vi "ConfMappIn.vi"(8 "error in (no error)":errorcluster, 11 "ConfMap In":string[](array[string])) -> (0 "error out":errorcluster, 1 "Discard?":bool, 3 "ConfMap Out":string[](array[string]))   [LabVIEW 2014, in "SeqLoop.lvlib"]
uses:
  SeqLoop.lvlib
panel:
  in  "Habilitada":bool
  in  "Bit":i32
  in  "Nro. Hardware":i32
  in  "Stop Med":bool
  in  "Add Med":bool
  in  "Descripción":string
  in  "Nro.":i32
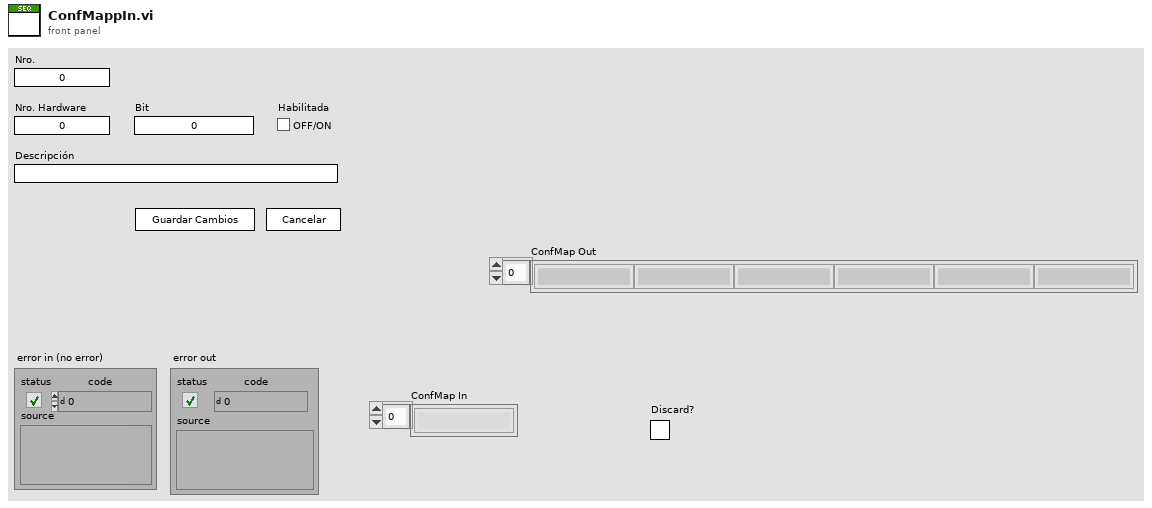
[diagram p1: front panel]
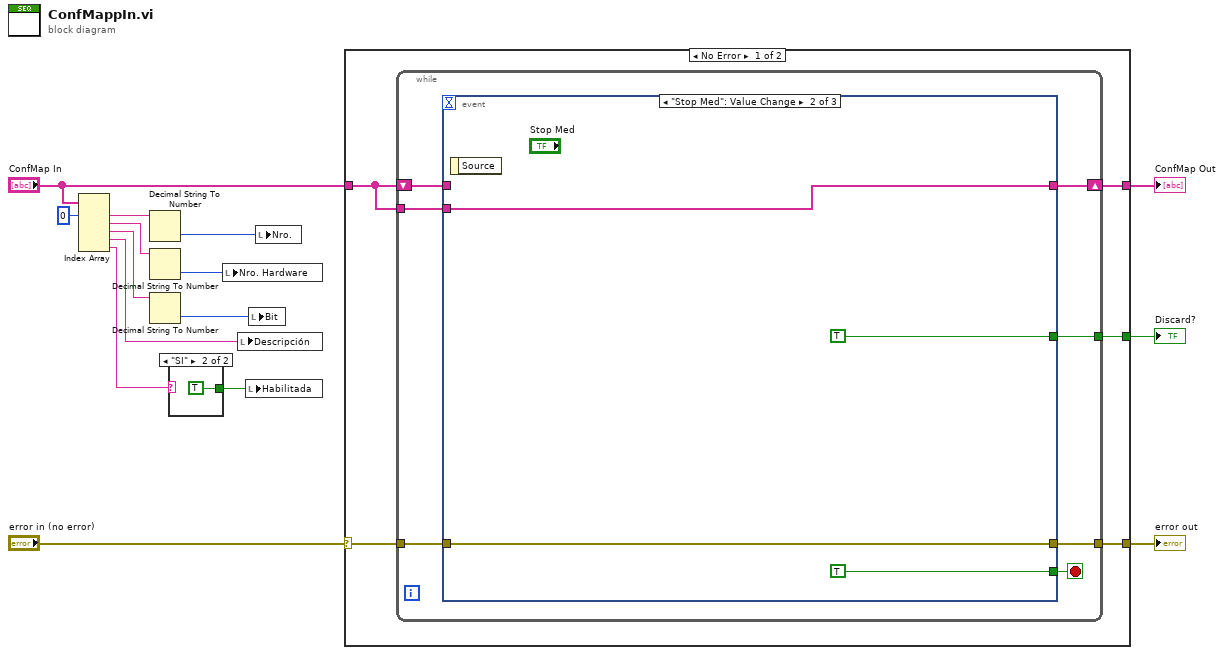
[diagram p0: block diagram]
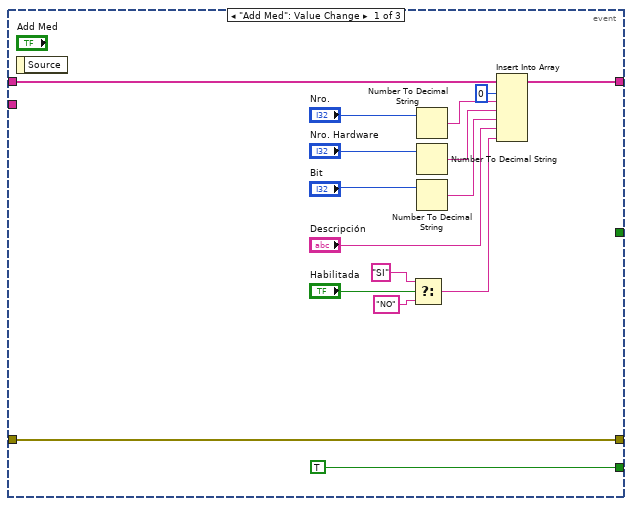
[diagram p3: hidden frame]
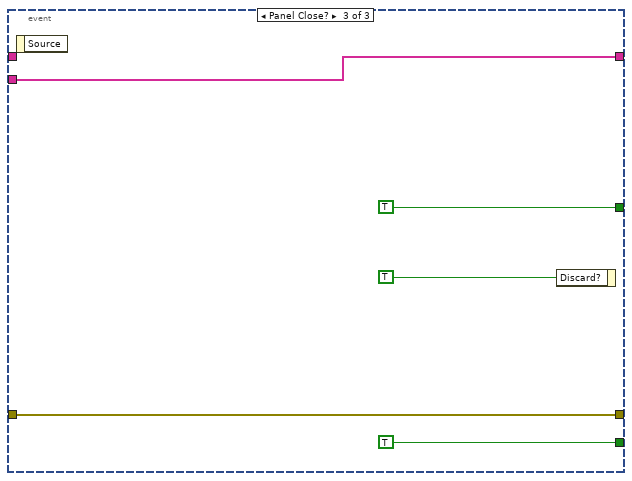
[diagram p4: hidden frame]
diagram:
  n1 = Index Array(array="ConfMap In", index #1=0 ("index")) -> (element #1=w10:string, element #2=w5:string, element #3=w4:string, element #4=w6:string, element #5=w3:string)  [unwired: 4 in]
  n2 = Decimal String To Number(string=w10) -> (number=w9:i32)  [unwired: 2 in, 1 out]
  n3 = Decimal String To Number(string=w5) -> (number=w8:i32)  [unwired: 2 in, 1 out]
  n4 = Decimal String To Number(string=w4) -> (number=w7:i32)  [unwired: 2 in, 1 out]
  n5 = case shown="\"SI\"" w3 {
    tunnel: [_ TRUE] -> w2
    frame "NO", Default {
    }
    frame "SI" {
    }
  }
  n6 = local write "Nro. Hardware"(w8) -> ()
  n7 = local write "Descripción"(w6) -> ()
  n8 = local write "Habilitada"(w2) -> ()
  n9 = local write "Bit"(w7) -> ()
  n10 = local write "Nro."(w9) -> ()
  n11 = case shown="No Error" "error in (no error)" {
    selector: "error in (no error)" -> [w19 w55]
    tunnel: [w21 w55] -> w14
    tunnel: "ConfMap In" -> [w18 w54]
    tunnel: [w20 w54] -> w13
    tunnel: [w17 _] -> w1
    frame No Error {
      n12 = while {
        tunnel: w19 -> [w27]
        tunnel: [w28] -> w21
        shift-right: [w24] -> w20
        shift-left: w18 -> [w25]
        tunnel: w18 -> [w23]
        tunnel: [w22] -> w17
        stop <- w26 stop-if-true
        n13 = event shown="[1] \"Stop Med\": Value Change" {
          selector: _ -> [_ _ _]
          dyn-events: _ -> [_ _ _]
          timeout: _ -> [_ _ _]
          tunnel: [w44 w47 w51] -> w28
          tunnel: w27 -> [w44 w47 w51]
          tunnel: [TRUE ("Discard?") TRUE ("Discard?") TRUE ("Discard?")] -> w26
          tunnel: w25 -> [w30 _ _]
          tunnel: [w36 w46 w50] -> w24
          tunnel: w23 -> [_ w46 w50]
          tunnel: [_ TRUE ("Discard?") TRUE ("Discard?")] -> w22
          event "Add Med": Value Change {
            n14 = event-data() -> ()  [unwired: 1 in, 1 out]
            n15 = Select(t="SI" ("Descripción 2"), s="Habilitada", f="NO" ("Descripción 2")) -> (s? t:f=w31:string)
            n16 = Number To Decimal String(number="Nro.") -> (decimal integer string=w35:string)  [unwired: 1 in]
            n17 = Number To Decimal String(number="Nro. Hardware") -> (decimal integer string=w34:string)  [unwired: 1 in]
            n18 = Number To Decimal String(number="Bit") -> (decimal integer string=w33:string)  [unwired: 1 in]
            n19 = Insert Into Array(array=w30, index=0, new element #1=w35, new element #2=w34, new element #3=w33, new element #4="Descripción", new element #5=w31) -> (w36:string[])
          }
          event "Stop Med": Value Change {
            n20 = event-data() -> ()  [unwired: 1 in, 1 out]
          }
          event Panel Close? {
            n21 = event-data() -> ()  [unwired: 1 in, 1 out]
            n22 = event-data("Discard?"=TRUE) -> ()  [unwired: 1 in, 1 out]
          }
        }
      }
    }
    frame Error {
    }
  }
  "error out" <- w14
  "ConfMap Out" <- w13
  "Discard?" <- w1
